vi "test_Study.vi"() -> ()   [LabVIEW 2023]
uses:
  Study/Study Actor/Study Actor/Study Actor.lvclass
  <vilib>/ni/Actors/Network Endpoint Actors/Protocols/Network Stream Strategy/Network Stream/Network Stream.lvclass/Network Stream.ctl
  <vilib>/ni/Actors/Network Endpoint Actors/Protocols/Network Stream Strategy/Network Stream Initiator/Network Stream Initiator.lvclass/Network Stream Initiator.ctl
  Study/Study Actor/Study Actor/Study Actor.lvclass/Study Actor.ctl
  DIO/DIO DAQmx Simulated CFGs/DO DAQmx PWM Fixed Freq CFG/DO DAQmx PWM Fixed Freq CFG.lvclass
  DIO/Virtual DIO/Virt PWM Fixed Freq Generator/Virt DAQmx Fixed Freq PWM Generator.lvclass
  Sample Series/Sample PWM Fans/Sample PWM Fans/Sample PWM Fans.lvclass
  Study/Study Actor/IStudy Actor Messages/Launch Series Msg/Launch Series Msg.lvclass/Launch Series Msg.ctl
  <vilib>/ActorFramework/Message Enqueuer/Message Enqueuer.lvclass/Message Enqueuer.ctl
  <vilib>/ni/Actors/Network Endpoint Actors/Protocols/Network Stream Strategy/Network Stream/Write Buffer Size.vi
  <vilib>/ni/Actors/Network Endpoint Actors/Protocols/Network Stream Strategy/Network Stream/Write Name.vi
  <vilib>/ActorFramework/Message Enqueuer/Enqueue.vi
  <vilib>/ni/Actors/Network Endpoint Actors/Protocols/Network Stream Strategy/Network Stream Initiator/Network Stream Initiator.lvclass
  <vilib>/MGI/Panel Manager/Panel/Window Position/Reference Position/Ref Top Level/Ref Top Level.lvclass
  Study/Study Actor/IStudy Actor Messages/Launch Series Msg/Launch Series Msg.lvclass
  <vilib>/ni/Actors/Network Endpoint Actors/Protocols/Network Stream Strategy/Network Stream/Write Address.vi
  <vilib>/MGI/Panel Manager/Panel/Window Position/Reference Position/Ref Top Level/Ref Top Level.vi
  <vilib>/MGI/Panel Manager/Panel Actor/Panel Actor/Launch Root Panel Window.vi
  <vilib>/Utility/LVClass/Get LV Class Name.vi
  <resource>/AFDebug/Generate Trace for Message.vi
  <vilib>/ActorFramework/Message Priority Queue/Priority Enqueue.vi
  <vilib>/MGI/Panel Manager/Panel Actor/Panel Actor/Panel Actor.lvclass
  <vilib>/MGI/Panel Manager/Panel/Panel.lvlib
  C:/Program Files/National Instruments/LabVIEW 2023/vi.lib/ni/Actors/Network Endpoint Actors/Protocols/Network Stream Strategy/Network Stream/Network Stream.lvclass
  C:/Program Files/National Instruments/LabVIEW 2023/vi.lib/ni/Actors/Network Endpoint Actors/Abstract Classes/Message Stream/Message Stream.lvclass
  C:/Program Files/National Instruments/LabVIEW 2023/vi.lib/ni/Actors/Network Endpoint Actors/Protocols/Network Stream Strategy/Network Stream Initiator/Network Stream Initiator.lvclass
  C:/Program Files/National Instruments/LabVIEW 2023/vi.lib/MGI/Panel Manager/Panel/Window Position/Reference Position/Reference Position.lvclass
  C:/Program Files/National Instruments/LabVIEW 2023/vi.lib/MGI/Panel Manager/Panel/Window Position/Window Position.lvclass
  C:/Program Files/National Instruments/LabVIEW 2023/vi.lib/MGI/Panel Manager/Panel/Window Position/Reference Position/Ref Top Level/Ref Top Level.lvclass
  C:/Program Files/National Instruments/LabVIEW 2023/vi.lib/MGI/Panel Manager/Panel Actor/Panel Actor/Panel Actor.lvclass
  C:/Program Files/National Instruments/LabVIEW 2023/vi.lib/ActorFramework/Actor/Actor.lvclass
  D:/git/HAL/HAL GOOP4/Study/Study Actor/Study Actor/Study Actor.lvclass
  D:/git/HAL/HAL GOOP4/Study/Study Actor/IStudy Actor/IStudy Actor.lvclass
  C:/Program Files/National Instruments/LabVIEW 2023/vi.lib/ni/Actors/Network Endpoint Actors/Nested Endpoint Caller/Nested Endpoint Caller/Nested Endpoint Caller.lvclass
panel:
  in  "Stop Button":bool
  out "Error Out":errorcluster
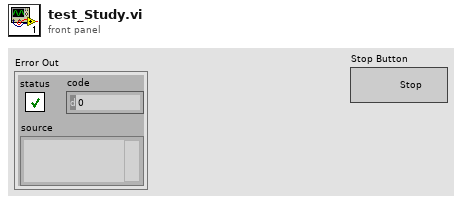
[diagram p1: front panel]
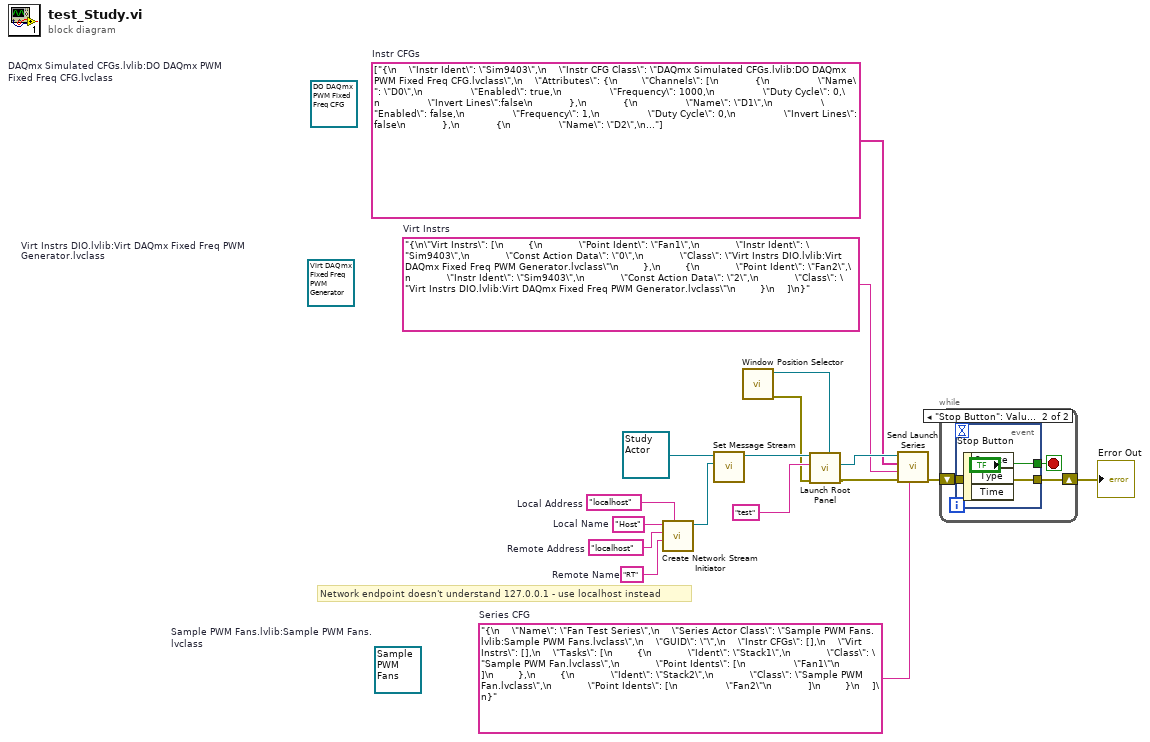
[diagram p0: block diagram]
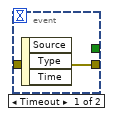
[diagram p2: hidden frame]
diagram:
  (unwired) refnum<class "Sample PWM Fans.lvclass"> refnum  # Sample PWM Fans.lvlib:Sample PWM Fans.lvclass
  (unwired) refnum<class "Virt DAQmx Fixed Freq PWM Generator.lvclass"> refnum  # Virt Instrs DIO.lvlib:Virt DAQmx Fixed Freq PWM Generator.lvclass
  (unwired) refnum<class "DO DAQmx PWM Fixed Freq CFG.lvclass"> refnum  # DAQmx Simulated CFGs.lvlib:DO DAQmx PWM Fixed Freq CFG.lvclass
  w3 = "{\n    \"Name\": \"Fan Test Series\",\n    \"Series Actor Class\": \"Sample PWM Fans.lvlib:Sample PWM Fans.lvclass\",\n    \"GUID\": \"\",\n    \"Instr CFGs\": [],\n    \"Virt Instrs\": [],\n    \"Tasks\": [\n        {\n            \"Ident\": \"Stack1\",\n            \"Class\": \"Sample PWM Fan.lvclass\",\n            \"Point Idents\": [\n                \"Fan1\"\n            ]\n        },\n        {\n            \"Ident\": \"Stack2\",\n            \"Class\": \"Sample PWM Fan.lvclass\",\n            \"Point Idents\": [\n                \"Fan2\"\n            ]\n        }\n    ]\n}"  # Series CFG
  w4 = "{\n\"Virt Instrs\": [\n        {\n            \"Point Ident\": \"Fan1\",\n            \"Instr Ident\": \"Sim9403\",\n            \"Const Action Data\": \"0\",\n            \"Class\": \"Virt Instrs DIO.lvlib:Virt DAQmx Fixed Freq PWM Generator.lvclass\"\n        },\n        {\n            \"Point Ident\": \"Fan2\",\n            \"Instr Ident\": \"Sim9403\",\n            \"Const Action Data\": \"2\",\n            \"Class\": \"Virt Instrs DIO.lvlib:Virt DAQmx Fixed Freq PWM Generator.lvclass\"\n        }\n    ]\n}"  # Virt Instrs
  w5 = string[] ["{\n    \"Instr Ident\": \"Sim9403\",\n    \"Instr CFG Class\": \"DAQmx Simulated CFGs.lvlib:DO DAQmx PWM Fixed Freq CFG.lvclass\",\n    \"Attributes\": {\n        \"Channels\": [\n            {\n                \"Name\": \"D0\",\n                \"Enabled\": true,\n                \"Frequency\": 1000,\n                \"Duty Cycle\": 0,\n                \"Invert Lines\":false\n            },\n            {\n                \"Name\": \"D1\",\n                \"Enabled\": false,\n                \"Frequency\": 1,\n                \"Duty Cycle\": 0,\n                \"Invert Lines\": false\n            },\n            {\n                \"Name\": \"D2\",\n                \"Enabled\": true,\n                \"Frequency\": 600,\n                \"Duty Cycle\": 0,\n                \"Invert Lines\": false\n            }\n        ],\n        \"Timing\": {\n            \"Type\" : \"Sample Clock\"\n            \"Samples per Channel\": 10000,\n            \"Sample Mode\": \"Continuous Samples\",\n            \"Sample Rate\": 100000,\n            \"Sample Clock Source\": \"OnboardClock\",\n            \"Active Edge\": \"Rising\"\n        },\n        \"Trigger\": {\n            \"Trigger Type\": \"No Trigger\"\n        },\n        \"Generation\": {\n            \"Regen Mode\": \"Allow Regeneration\"\n        }\n    }\n}"]  # Instr CFGs
  w10 = "RT"  # Remote Name
  w9 = "localhost"  # Local Address
  w11 = "localhost"  # Remote Address
  w12 = "Host"  # Local Name
  # "Network endpoint doesn't understand 127.0.0.1 - use localhost instead"
  n1 = call <vilib>:"Create Network Stream Initiator.vi"("Local Address"=w9, "Remote Name"=w10, "Remote Address"=w11, "Name"=w12) -> ("Network Stream Initiator out"=w8:refnum<class "Network Stream Initiator.lvclass">)  [unwired: 7 in]
  n2 = call "Set Message Stream.vi"("Message Stream.lvclass"=w8, "Study Actor in"=refnum<class "Study Actor.lvclass"> refnum ("HAL GOOP4.lvlib:Study Actor.lvlib:Study Actor.lvclass")) -> ("Study Actor out"=w13:refnum<class "Study Actor.lvclass">)  [unwired: 9 in]
  n3 = call-poly <vilib>:"Window Position Selector.vi"() -> ("Error Out"=w6:errorcluster, "Ref Top Level out"=w16:refnum<class "Ref Top Level.lvclass">)  [unwired: 10 in]
  n4 = call-poly <vilib>:"Launch Root Panel.vi"("Window Position (Maximize First Call)"=w16, "Error In"=w6, "Title"="test", "Panel Actor in"=w13) -> ("Error Out"=w15:errorcluster, "Actor's Enqueuer"=w7:refnum<class "Message Enqueuer.lvclass">)  [unwired: 6 in]
  n5 = call "Send Launch Series.vi"("Series CFG"=w3, "error in (no error)"=w15, "Virt Instrs"=w4, "Instr CFGs"=w5, "Message Enqueuer"=w7) -> ("error out"=w2:errorcluster)  [unwired: 5 in, 1 out]
  n6 = while {
    shift-right: [w18] -> w1
    shift-left: w2 -> [w20]
    stop <- w19 stop-if-true
    n7 = event shown="[1] \"Stop Button\": Value Change" {
      selector: _ -> [_ _]
      dyn-events: _ -> [_ _]
      timeout: _ -> [_ _]
      tunnel: w20 -> [w21 w22]
      tunnel: [w21 w22] -> w18
      tunnel: [_ "Stop Button"] -> w19
      event Timeout {
        n8 = event-data() -> ()  [unwired: 1 in, 3 out]
      }
      event "Stop Button": Value Change {
        n9 = event-data() -> ()  [unwired: 1 in, 3 out]
      }
    }
  }
  "Error Out" <- w1
